vi "Write Meter Measurement DVR.vi"(8 "error in":errorcluster, 10 "Meter_Measurement":T1, 11 "EMS Generic in":refnum<class "EMS Generic.lvclass">) -> (0 "error out":errorcluster, 3 "EMS Generic out":refnum<class "EMS Generic.lvclass">)   [LabVIEW 2018, in "EMS Generic Actor.lvlib" / "EMS Generic.lvclass"]
uses:
  EMS Generic.lvclass
  <vilib>/ORNL/CSEISMIC DDS/CSEISMIC DDS Base/Data Types/Meter_Measurement.ctl
  <vilib>/ORNL/CSEISMIC DDS/CSEISMIC DDS Base/Data Types/Controls/DeviceID.ctl
  EMS Generic.lvclass/EMS Generic.ctl
  <vilib>/ORNL/CSEISMIC DDS/CSEISMIC DDS Base/CSEISMIC DDS.lvclass
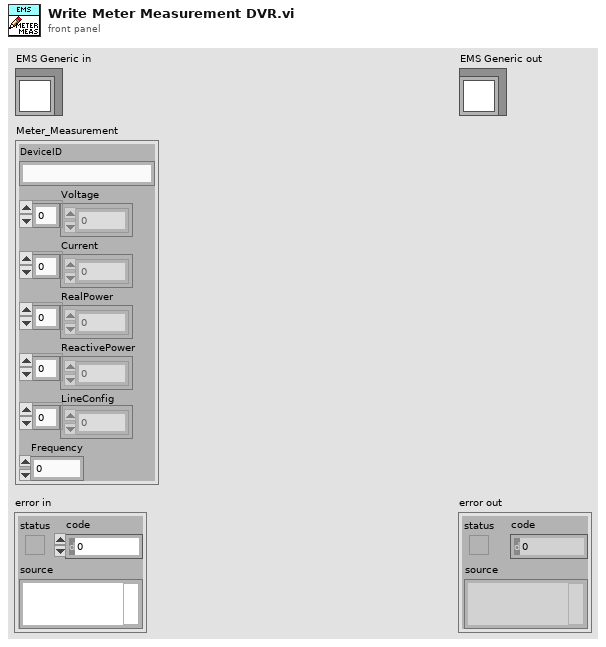
[diagram p1: front panel]
types:
  T1 = typedef "CSEISMIC DDS.lvlib/CSEISMIC DDS.lvclass/Meter_Measurement.ctl" = cluster{"DeviceID":T2, "Voltage":dbl[], "Current":dbl[], "RealPower":dbl[], "ReactivePower":dbl[], "LineConfig":u8[], "Frequency":dbl}
  T2 = typedef "CSEISMIC DDS.lvlib/CSEISMIC DDS.lvclass/DeviceID.ctl" = string
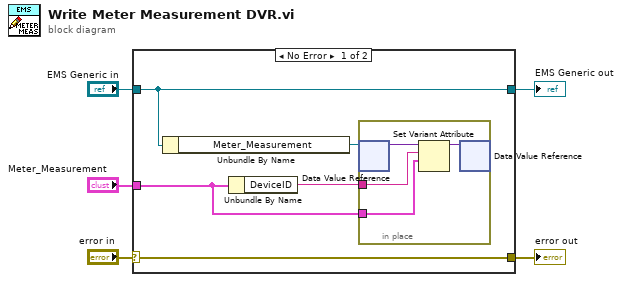
[diagram p0: block diagram]
diagram:
  n1 = case shown="No Error" "error in" {
    selector: "error in" -> [w10 w16]
    tunnel: [w10 w16] -> w4
    tunnel: [w9 w15] -> w2
    tunnel: "EMS Generic in" -> [w9 w15]
    tunnel: "Meter_Measurement" -> [w7 _]
    frame No Error {
      n2 = Unbundle By Name(w9) -> ("Meter_Measurement"=w6:refnum<data-value>)
      n3 = Unbundle By Name(w7) -> ("DeviceID"=w8:T2)
      n4 = in-place {
        in-place-border: w8 -> [w12]
        in-place-border: w7 -> [w11]
        n5 = in-place-dvr #1(w6) -> (w14:variant)  [unwired: 1 out]
        n6 = Set Variant Attribute(Variant=w14, name=w12, value=w11) -> (Variant out=w13:variant)  [unwired: 1 in, 2 out]
        n7 = in-place-dvr #1(w13) -> ()  [unwired: 2 out]
      }
    }
    frame Error {
    }
  }
  "error out" <- w4
  "EMS Generic out" <- w2
